vi "setREFfilterConfig.vi"(8 "error in (no error)":errorcluster, 10 "REF filter":T1={"TC (s)"=0.3, "order"=2} {"TC (s)" format="%#_6p"}, 11 "Instrument.Lockin in":refnum<class "Instrument.Lockin.lvclass">) -> (0 "error out":errorcluster, 3 "Instrument.Lockin out":refnum<class "Instrument.Lockin.lvclass">)   [LabVIEW 2016, in "Instrument.Lockin.lvclass"]
doc: "API to configure the REF.\n\nIf address=\"\", this API reads from localhost\nIf address is remote lockin, you need to add this computer to allowed whitelist on the lockin computer you are trying to access."
uses:
  Instrument.Lockin.lvclass
  LockinDAQ/Typedefs/REF filter-cluster.ctl
  Typedefs/Instrument.Lockin.Commands--Enum.ctl
  LockinDAQ/LockinDAQ.lvclass
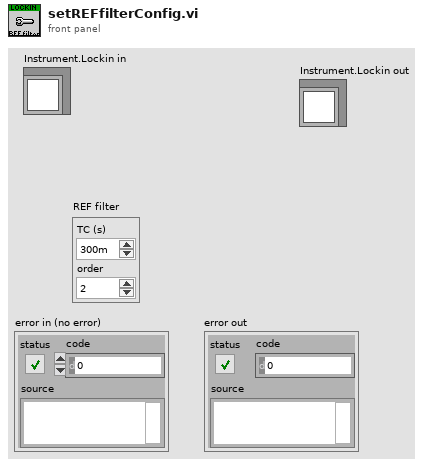
[diagram p1: front panel]
types:
  T1 = typedef "LockinDAQ.lvclass/REF filter-cluster.ctl" = cluster{"TC (s)":dbl, "order":i32}
  T2 = typedef "Instrument.Lockin.lvclass/Instrument.Lockin.Commands--Enum.ctl" = enum16{"configAO", "configAO_Amplitude", "configAO_DC", "configAO_Frequency", "configAO_Phase", "configAO_Function", "configAO_I+", "configREF", "configREF_Frequency", "configREF_Phase", "configREF_Filter", "configIVmode", "Reset", "configSampling", "Trigger", "getAO", "getAI", "getResults", "getTrigger", "getIVmode", "getSampling", "getAOconfig", "getREFconfig", "getREF_Filter", "configGain", "getGain", "configAutoSampling", "getAutoSampling", "configSweep", "configSweepFile", "getStatus", "getSweepResults", "startSweep", "stopSweep"}
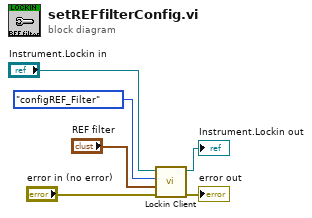
[diagram p0: block diagram]
diagram:
  n1 = call "Lockin Client.vi"("error in (no error)"="error in (no error)", "Data"="REF filter", "Command"=Instrument.Lockin.Commands--Enum."configREF_Filter", "Instrument.Lockin in"="Instrument.Lockin in") -> ("error out"=→"error out":errorcluster, "Instrument.Lockin out"=→"Instrument.Lockin out":refnum<class "Instrument.Lockin.lvclass">)  [unwired: 5 in, 1 out]
